vi "LittleTiming.vi"(1 "Intent":bool, 2 "Override":bool, 3 "FPGA Time":dbl, 4 "Limit Switch Pressed":bool) -> (0 "Motor Speed out":dbl)   [LabVIEW 2013]
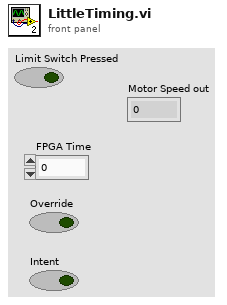
[diagram p1: front panel]
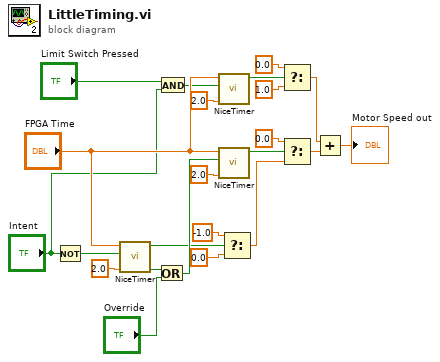
[diagram p0: block diagram]
diagram:
  n1 = Not(x="Intent") -> (.not. x?=w23:bool)
  n2 = call "NiceTimer.vi"("Wait Duration"=2.0, "Reset Timer"=w23, "Current time"="FPGA Time") -> ("Single Event True"=w20:bool, "Time's up bubby"=w17:bool)  [unwired: 7 in]
  n3 = Or(x=w20, y="Override") -> (x .or. y?=w21:bool)
  n4 = And(x="Limit Switch Pressed", y="Intent") -> (x .and. y?=w3:bool)
  n5 = call "NiceTimer.vi"("Wait Duration"=2.0, "Reset Timer"=w3, "Current time"="FPGA Time") -> ("Time's up bubby"=w7:bool)  [unwired: 7 in, 1 out]
  n6 = call "NiceTimer.vi"("Wait Duration"=2.0, "Reset Timer"=w21, "Current time"="FPGA Time") -> ("Time's up bubby"=w13:bool)  [unwired: 7 in, 1 out]
  n7 = Select(t=-1.0 ("f"), s=w17, f=0.0) -> (s? t:f=w14:dbl)
  n8 = Select(t=0.0, s=w7, f=1.0 ("t")) -> (s? t:f=w9:dbl)
  n9 = Select(t=0.0, s=w13, f=w14) -> (s? t:f=w10:dbl)
  n10 = Add(x=w9, y=w10) -> (x+y=→"Motor Speed out":dbl)
